vi "test.vi"() -> ()   [LabVIEW 2013]
panel:
  in  "Numeric":dbl
  in  "MG17Motor":refnum<k7>(container)
  in  "stop":bool
  in  "Serial":i32=90848557
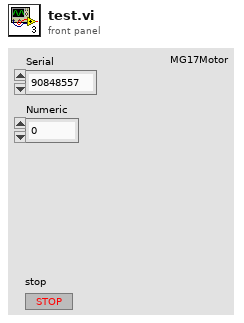
[diagram p1: front panel]
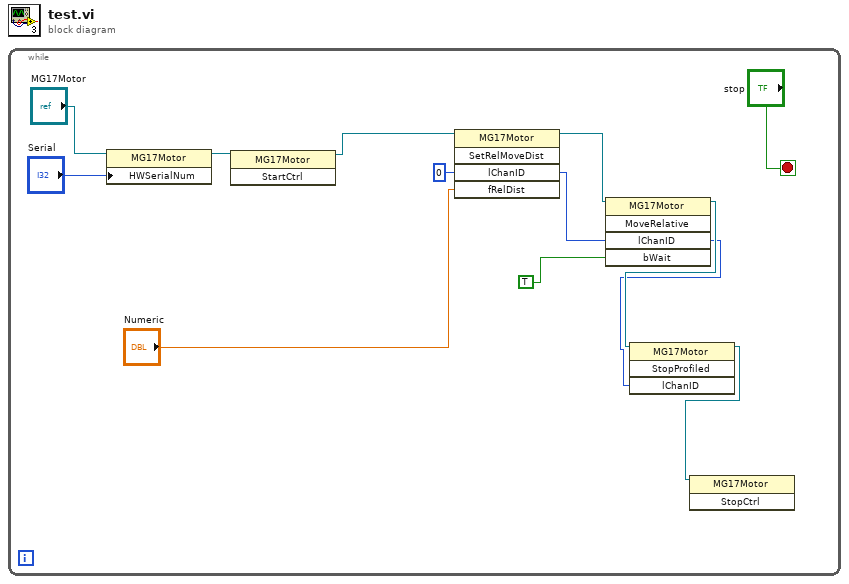
[diagram p0: block diagram]
diagram:
  n1 = while {
    stop <- "stop" stop-if-true
    n2 = property class="MG17Motor"(reference="MG17Motor", "HWSerialNum"="Serial") -> (reference out=w12:refnum<k7>)  [unwired: 1 in, 1 out]
    n3 = invoke class="MG17Motor" method="StartCtrl"(reference=w12) -> (reference out=w9:refnum<k7>)  [unwired: 2 in, 2 out]
    n4 = invoke class="MG17Motor" method="SetRelMoveDist"(reference=w9, "lChanID"=0, "fRelDist"="Numeric") -> (reference out=w6:refnum<k7>, "lChanID"=w7:i32)  [unwired: 2 in, 3 out]
    n5 = invoke class="MG17Motor" method="MoveRelative"(reference=w6, "lChanID"=w7, "bWait"=TRUE) -> (reference out=w5:refnum<k7>, "lChanID"=w3:i32)  [unwired: 2 in, 3 out]
    n6 = invoke class="MG17Motor" method="StopProfiled"(reference=w5, "lChanID"=w3) -> (reference out=w4:refnum<k7>)  [unwired: 2 in, 3 out]
    n7 = invoke class="MG17Motor" method="StopCtrl"(reference=w4) -> ()  [unwired: 2 in, 3 out]
  }
